vi "Create.vi"(8 "error in (no error)":errorcluster, 11 "count (1)":u64=1) -> (0 "error out":errorcluster, 3 "status pointer":refnum<class "Status Pointer.lvclass">)   [LabVIEW 2020, in "DSF Core.lvlib" / "Status Pointer.lvclass"]
uses:
  Status Pointer.lvclass
  C:/Program Files (x86)/National Instruments/LabVIEW 2020/vi.lib/NI/Memory Manager/Classes/Pointer/Pointer.lvclass
  Status Data.ctl
  <vilib>/NI/Memory Manager/Classes/Pointer/Pointer.lvclass/Pointer.ctl
  <vilib>/NI/Memory Manager/Classes/Pointer/Set Address.vi
  <vilib>/NI/Memory Manager/Classes/Pointer/Set Size.vi
  <vilib>/NI/Memory Manager/Classes/Pointer/Set Internal.vi
  <vilib>/NI/Memory Manager/Classes/Pointer/Get Address.vi
  <vilib>/NI/Memory Manager/Classes/Pointer/Check Size.vi
  <vilib>/NI/Memory Manager/Classes/Pointer/Check Null Pointer.vi
  <vilib>/NI/Memory Manager/Classes/Pointer/Errors.vi
  <vilib>/NI/Memory Manager/Classes/Pointer/Out of Bounds.vi
  <vilib>/NI/Memory Manager/Classes/Pointer/Get Size.vi
  <vilib>/NI/Memory Manager/Classes/Pointer/Null Pointer.vi
  <vilib>/NI/Memory Manager/Classes/Pointer/Is Null.vi
  <vilib>/NI/Memory Manager/VIs/Write String to Source.vi
  <vilib>/NI/Memory Manager/Classes/Pointer/Write Pointer Size to Error.vi
  <vilib>/NI/Memory Manager/Classes/Pointer/Create Error.vi
  <vilib>/NI/Memory Manager/VIs/Write Numeric to Source.vi
  <vilib>/NI/Memory Manager/VIs/Write Numeric Scalar to Source (Base10 U64).vi
  <vilib>/NI/Memory Manager/VIs/New Error Cluster.vi
  <vilib>/NI/Memory Manager/VIs/New Error Cluster (512B).vi
  <vilib>/NI/Memory Manager/VIs/Set Error Status.vi
  <vilib>/NI/Memory Manager/VIs/Set Error Code.vi
  <vilib>/NI/Memory Manager/VIs/Set Error Source.vi
  <vilib>/NI/Memory Manager/Constants/Constants.vi
  <vilib>/NI/Memory Manager/Constants/Library Name.vi
  <vilib>/NI/Memory Manager/Classes/Pointer/Pointer Error Info.vi
  <vilib>/NI/Memory Manager/Constants/Pointer Class Name.vi
  <vilib>/NI/Memory Manager/Classes/Pointer/Pointer.lvclass
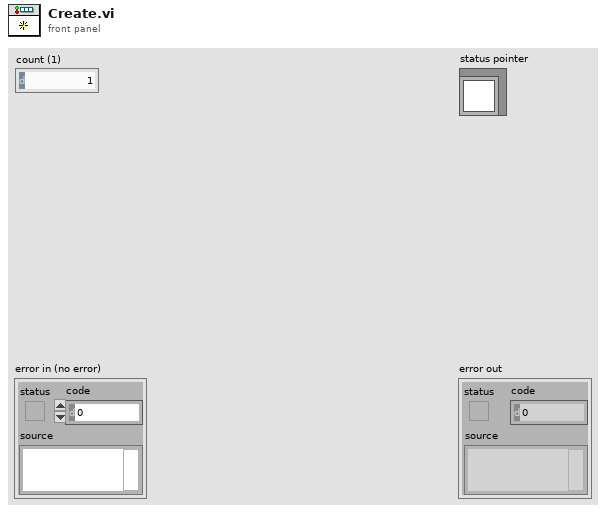
[diagram p1: front panel]
types:
  T1 = typedef "DSF Core.lvlib/Status Pointer.lvclass/Status Data.ctl" = cluster{"duration":u64, "period":u64, "iteration":u64, "late count":u64}
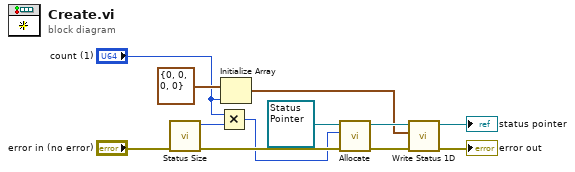
[diagram p0: block diagram]
diagram:
  n1 = call "Status Size.vi"("error in (no error)"="error in (no error)") -> ("error out"=w5:errorcluster, "size"=w8:u64)  [unwired: 9 in]
  n2 = Multiply(x="count (1)", y=w8) -> (x*y=w1:u64)
  n3 = Initialize Array(T1 {"duration"=0, "period"=0, "iteration"=0, "late count"=0} ("Transfer Group status"), "count (1)") -> (w2:T1[])
  n4 = call <vilib>:"Allocate.vi"("error in (no error)"=w5, "size"=w1, "Pointer type"=refnum<class "Status Pointer.lvclass"> refnum ("Transfer Group Status in")) -> ("error out"=w4:errorcluster, "Pointer out"=w3:refnum<class "Status Pointer.lvclass">)  [unwired: 7 in]
  n5 = call "Write Status 1D.vi"("error in (no error)"=w4, "statuses"=w2, "status pointer in"=w3) -> ("error out"=→"error out":errorcluster, "status pointer out"=→"status pointer":refnum<class "Status Pointer.lvclass">)  [unwired: 7 in]
